vi "IMAQ Image Array to KLB File.vi"(8 "error in (no error)":errorcluster, 9 "path":path, 10 "KLB Settings":T1={"Logical Cores"=enum."4", "pixelSize (um)"=[1.0, 1.0, 1.0, 1.0, 1.0], "blockSize"=[96, 96, 8, 1, 1], "compressionType"=enum."BZip2", "metadata"=""} {"pixelSize (um)" min=0.01 max=10 step=0.01 format="%.2f"}, 11 "Images to Compress":T4[](array[typedef])) -> (0 "error out":errorcluster, 4 "elapsed (ms)":u32)   [LabVIEW 2013, in "KLB.lvlib"]
doc: "Writes IMAQ image array to KLB file with no restrictions.\n\nUses write KLB stack slices\n\nImages that have no boarder or buffer are passed using IMAQ pointer\n\nImages that have extra space need trimed using a modified version of IMAQ Stack to 1D Array.vi then passed by pointer per image. (Whole stack not converted to one pointer)\n\nInputs\n\n(Required) Images to compress - Pointers to IMAQ images\n(Required) Path - Full path and filename to create for KLB File\n\n(Recommended) KLB Settings - Logicals Cores, pixelSize, blockSize, compressionType, metadata\n Logicals Cores - Allows you to pick how much cpu power to toss at compression \n default (4)\n pixelSize - float32 pixelSize [5]: sampling of each dimension (in units of µm, index count, seconds)\n default (1,1,1,1,1)\n blockSize - uint32 blockSize [5]: block size used to partition the data in each dimension\n default (96,96,8,1,1)\n compressionType - Pick the type of compression\n default (BZip2)\n metadata - char metadata [256]: character block providing space for user-defined metadata\n default (\"\")"
uses:
  KLB.lvlib
  <vilib>/vision/Image Controls.llb/IMAQ Image.ctl
  Type Defs/KLB Settings Cluster.ctl
  Type Defs/KLB # of CPUs enum.ctl
  Type Defs/KLB compression type enum.ctl
  klb.dll
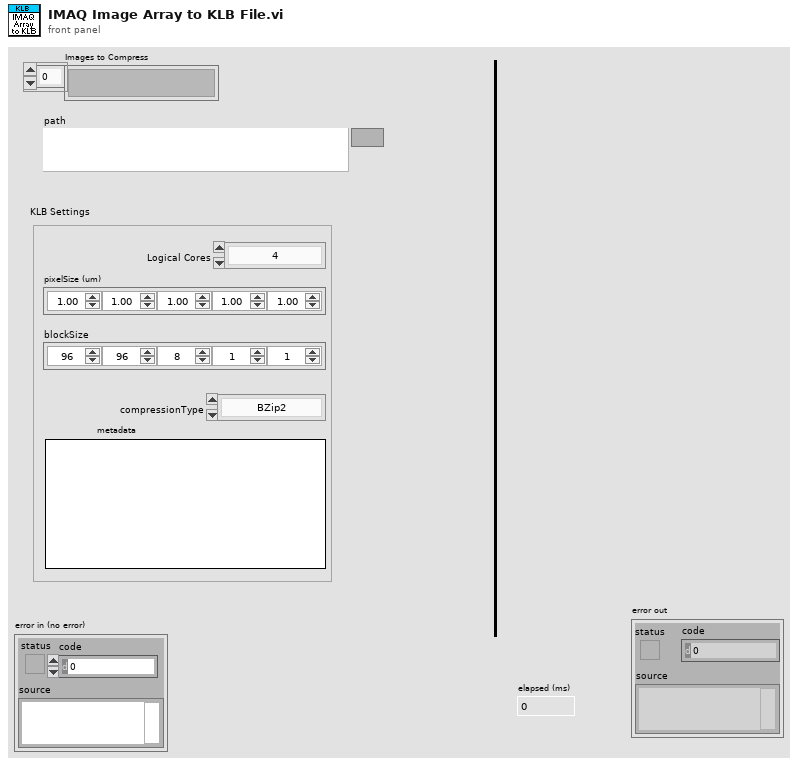
[diagram p1: front panel]
types:
  T1 = typedef "KLB.lvlib/KLB Settings Cluster.ctl" = cluster{"Logical Cores":T2, "pixelSize (um)":sgl[], "blockSize":u32[], "compressionType":T3, "metadata":string}
  T2 = typedef "KLB.lvlib/KLB # of CPUs enum.ctl" = enum16{"CPU 25%", "CPU 50%", "CPU 75%", "CPU All but 1", "1", "4", "8", "16"}
  T3 = typedef "KLB.lvlib/KLB compression type enum.ctl" = enum8{"Uncompressed", "BZip2"}
  T4 = typedef "IMAQ Image.ctl" = refnum<image>
  T5 = enum32{"Map Pixel Pointer", "Unmap Pixel Pointer", "Get Pixels Infos"}
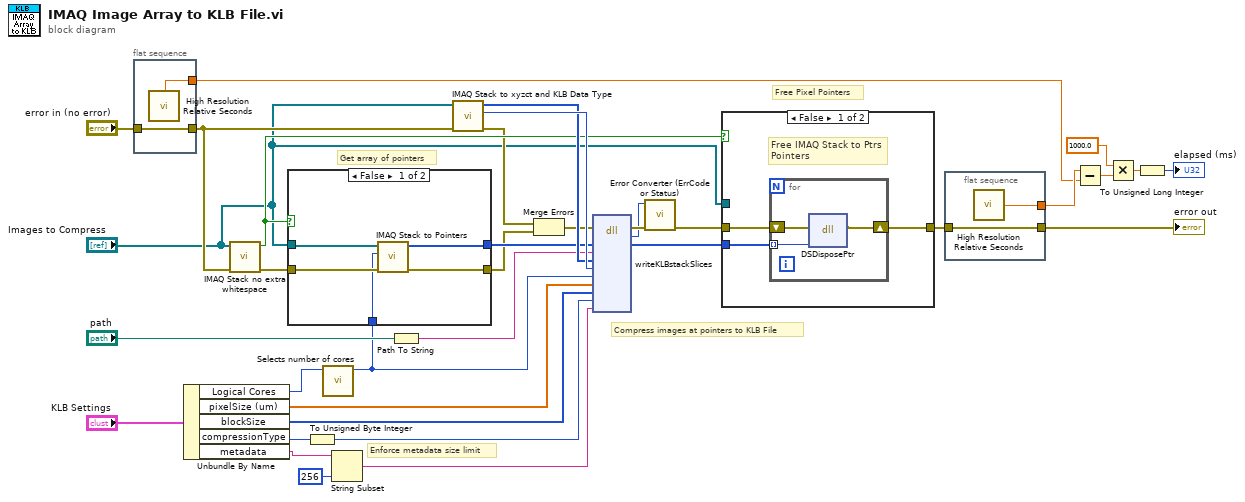
[diagram p0: block diagram]
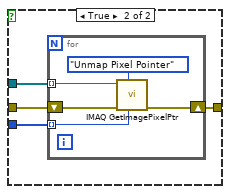
[diagram p2: hidden frame]
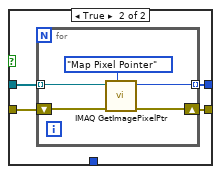
[diagram p3: hidden frame]
diagram:
  # "Compress images at pointers to KLB File"
  # "Get array of pointers"
  # "Enforce metadata size limit"
  # "Free Pixel Pointers"
  n1 = flat-sequence {
    tunnel: "error in (no error)" -> [w37]
    tunnel: [w37] -> w33
    tunnel: [w36] -> w14
    frame #0 {
      n2 = call <vilib>:"High Resolution Relative Seconds.vi"() -> ("relative seconds"=w36:dbl)
    }
  }
  n3 = Unbundle By Name("KLB Settings") -> ("Logical Cores"=w21:T2, "pixelSize (um)"=w20:sgl[], "blockSize"=w19:u32[], "compressionType"=w9:T3, "metadata"=w7:string)
  n4 = call "IMAQ Stack no extra whitespace"("error in"=w33, "Images to Compress"="Images to Compress") -> ("error out"=w2:errorcluster, "No Whitespace"=w32:bool)  [unwired: 8 in]
  n5 = To Unsigned Byte Integer(number=w9) -> (unsigned 8bit integer=w8:u8)
  n6 = call "Selects number of cores.vi"("Logical cores"=w21) -> ("Number of logical cores to use"=w1:i32)  [unwired: 10 in]
  n7 = case shown="False" w32 {
    tunnel: [w39 w46] -> w31
    tunnel: [w38 w45] -> w28
    tunnel: "Images to Compress" -> [w41 w44]
    tunnel: w2 -> [w42 w43]
    tunnel: w1 -> [w40 _]
    frame False {
      n8 = call "IMAQ Stack to Pointers.vi"("error in"=w42, "Number of threads"=w40, "IMAQ Image Array"=w41) -> ("error out"=w38:errorcluster, "Pointers Out"=w39:u64[])  [unwired: 7 in]
    }
    frame True {
      n9 = for {
        tunnel: w44 -> [w47] mode=indexing
        tunnel: [w50] -> w46 mode=indexing
        shift-right: [w48] -> w45
        shift-left: w43 -> [w49]
        n10 = call "IMAQ GetImagePixelPtr"("Function"=T5."Map Pixel Pointer", "error in (no error)"=w49, "Image"=w47) -> ("error out"=w48:errorcluster, "Pixel Pointer out"=w50:u64)  [unwired: 3 in, 4 out]
      }
    }
  }
  n11 = String Subset(string=w7, length (rest)=256 ("length (rest)")) -> (substring=w5:string)  [unwired: 1 in]
  n12 = Path To String(path="path") -> (string=w29:string)
  n13 = call "IMAQ Stack to xyzct and KLB Data Type.vi"("error in"=w33, "IMAQ Stack"="Images to Compress") -> ("error out"=w26:errorcluster, "KLB Data Type"=w35:u8, "XYZCT"=w34:u32[])  [unwired: 7 in]
  n14 = Merge Errors(w26, w28) -> (w27:errorcluster)
  n15 = dll-call lib="C:/Users/achiu/Documents/Projects - Current/HHMI - WBA/fpga_wba_repo/WBA 8 Tap 8-bit sector/Host/File IO/KLB/klb.*" fn="writeKLBstackSlices"(error in=w27, "im"=w31, "filename"=w29, "xyzct"=w34, "dataType"=w35, "numThreads"=w1, "pixelSize"=w20, "blockSize"=w19, "compressionType"=w8, "metadata"=w5) -> (error out=w25:errorcluster, "return type"=w24:i32, "im"=w4:u64[])  [unwired: 10 in, 1 out]
  n16 = call "Error Converter (ErrCode or Status).vi"("error in (no error)"=w25, "error code"=w24) -> ("error out"=w23:errorcluster)  [unwired: 9 in]
  n17 = case shown="False" w32 {
    tunnel: w23 -> [w53 w61]
    tunnel: "Images to Compress" -> [_ w60]
    tunnel: [w52 w59] -> w17
    tunnel: w4 -> [w54 w58]
    frame False {
      # "Free IMAQ Stack to Ptrs\nPointers"
      n18 = for {
        tunnel: w54 -> [w57] mode=indexing
        shift-right: [w55] -> w52
        shift-left: w53 -> [w56]
        n19 = dll-call lib="LabVIEW" fn="DSDisposePtr"(error in=w56, "Pointer"=w57) -> (error out=w55:errorcluster)  [unwired: 4 in, 1 out]
      }
    }
    frame True {
      n20 = for {
        shift-right: [w64] -> w59
        shift-left: w61 -> [w65]
        tunnel: w60 -> [w63] mode=indexing
        tunnel: w58 -> [w62] mode=indexing
        n21 = call "IMAQ GetImagePixelPtr"("Pixel Pointer in"=w62, "Function"=T5."Unmap Pixel Pointer", "error in (no error)"=w65, "Image"=w63) -> ("error out"=w64:errorcluster)  [unwired: 2 in, 5 out]
      }
    }
  }
  n22 = flat-sequence {
    tunnel: w17 -> [w68]
    tunnel: [w68] -> w16
    tunnel: [w67] -> w15
    frame #0 {
      n23 = call <vilib>:"High Resolution Relative Seconds.vi"() -> ("relative seconds"=w67:dbl)
    }
  }
  n24 = Subtract(x=w15, y=w14) -> (x-y=w13:dbl)
  n25 = Multiply(x=1000.0, y=w13) -> (x*y=w11:dbl)
  n26 = To Unsigned Long Integer(number=w11) -> (unsigned 32bit integer=→"elapsed (ms)":u32)
  "error out" <- w16
